vi "ConvertTimes - Single.vi"(1 "GP22 Output":u32) -> (0 "Time/s":dbl)   [LabVIEW 2017, in "GP22_TDC_Arduinoed.lvlib"]
doc: "Convert fixed point output of GP22 to time value in seconds. \n\nDepending on whether the TDC is in calibration mode or not, adjust the raw data by either the Ref clock's period (calibrated mode) or the calibration LSB time (uncalibrated mode)."
uses:
  GP22_TDC_Arduinoed.lvlib
  Public/Globals.vi
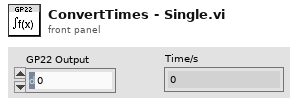
[diagram p1: front panel]
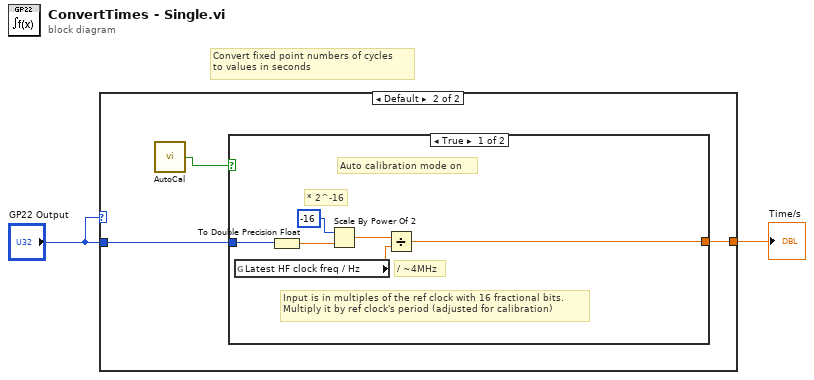
[diagram p0: block diagram]
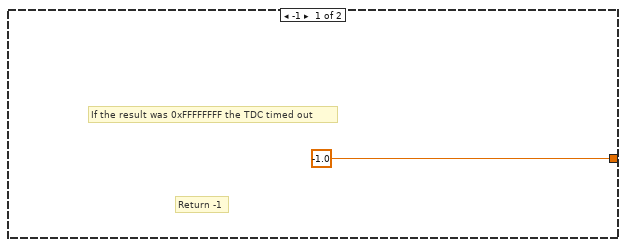
[diagram p2: hidden frame]
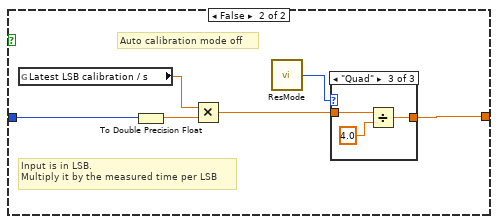
[diagram p3: hidden frame]
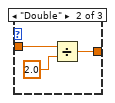
[diagram p5: hidden frame]
diagram:
  # "Convert fixed point numbers of cycles\nto values in seconds"
  n1 = case shown="Default" "GP22 Output" {
    tunnel: [-1.0 w6] -> w2
    tunnel: "GP22 Output" -> [_ w5]
    frame -1 {
      # "Return -1"
      # "If the result was 0xFFFFFFFF the TDC timed out"
    }
    frame Default {
      n2 = call "AutoCal.vi"() -> ("Autocal mode?"=w4:bool)  [unwired: 2 in]
      n3 = case shown="True" w4 {
        tunnel: [w11 w15] -> w6
        tunnel: w5 -> [w9 w18]
        frame True {
          # "Input is in multiples of the ref clock with 16 fractional bits.\nMultiply it by ref clock's period (adjusted for calibration)"
          # "/ ~4MHz"
          # "Auto calibration mode on"
          # "* 2^-16"
          n4 = global read "Globals.vi" "Latest HF clock freq / Hz"() -> (w7:dbl)
          n5 = To Double Precision Float(number=w9) -> (double precision float=w8:dbl)
          n6 = Scale By Power Of 2(n=i16 -16, x=w8) -> (x*2^n=w12:dbl)
          n7 = Divide(x=w12, y=w7) -> (x/y=w11:dbl)
        }
        frame False {
          # "Input is in LSB. \nMultiply it by the measured time per LSB"
          # "Auto calibration mode off"
          n8 = global read "Globals.vi" "Latest LSB calibration / s"() -> (w16:dbl)
          n9 = To Double Precision Float(number=w18) -> (double precision float=w17:dbl)
          n10 = Multiply(x=w16, y=w17) -> (x*y=w14:dbl)
          n11 = call "ResMode.vi"() -> ("Resolution mode"=w13:enum16{"Single", "Double", "Quad"})  [unwired: 2 in]
          n12 = case shown="\"Quad\"" w13 {
            tunnel: [w19 w22 w25] -> w15
            tunnel: w14 -> [w19 w21 w24]
            frame "Single" {
            }
            frame "Double" {
              n13 = Divide(x=w21, y=2.0) -> (x/y=w22:dbl)
            }
            frame "Quad" {
              n14 = Divide(x=w24, y=4.0) -> (x/y=w25:dbl)
            }
          }
        }
      }
    }
  }
  "Time/s" <- w2
